vi "wait.vi"(8 "error in (no error)":errorcluster, 10 "wait for":T1, 11 "DL090430TriggeredExperimentController in":refnum<class "ExperimentControllerDL090430DAQmxTriggered.lvclass">) -> (0 "error out":errorcluster, 2 "experiment finished?":bool, 3 "DL090430TriggeredExperimentController out":refnum<class "ExperimentControllerDL090430DAQmxTriggered.lvclass">)   [LabVIEW 2010, in "ExperimentControllerDL090430DAQmxTriggered.lvclass"]
uses:
  ExperimentControllerDL090430DAQmxTriggered.lvclass
  wait_for_enum.ctl
  ExperimentControllerDL090430DAQmxTriggered.lvclass/ExperimentControllerDL090430DAQmxTriggered.ctl
  <vilib>/DAQmx/read.llb/DAQmx Read (Analog DBL 1Chan 1Samp).vi
  <vilib>/DAQmx/configure/trigger.llb/DAQmx Start Trigger (Digital Edge).vi
  <vilib>/daqmx/miscellaneous.llb/DAQmx Fill In Error Info.vi
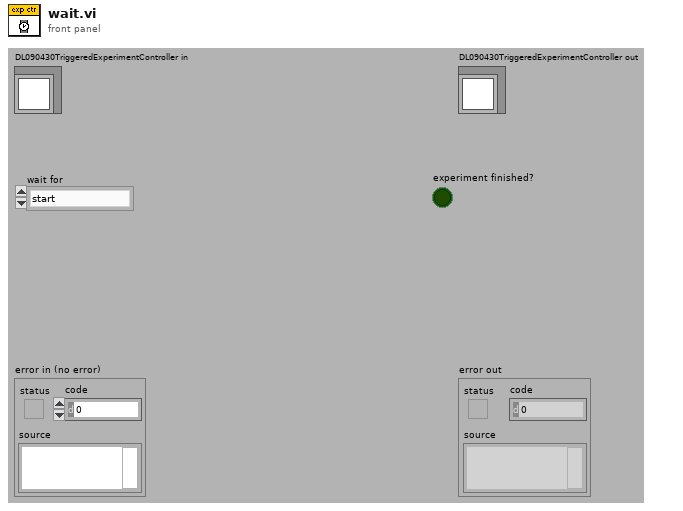
[diagram p1: front panel]
types:
  T1 = typedef "ExperimentControllerDL090430DAQmxTriggered.lvclass/wait_for_enum.ctl" = enum16{"start", "stop"}
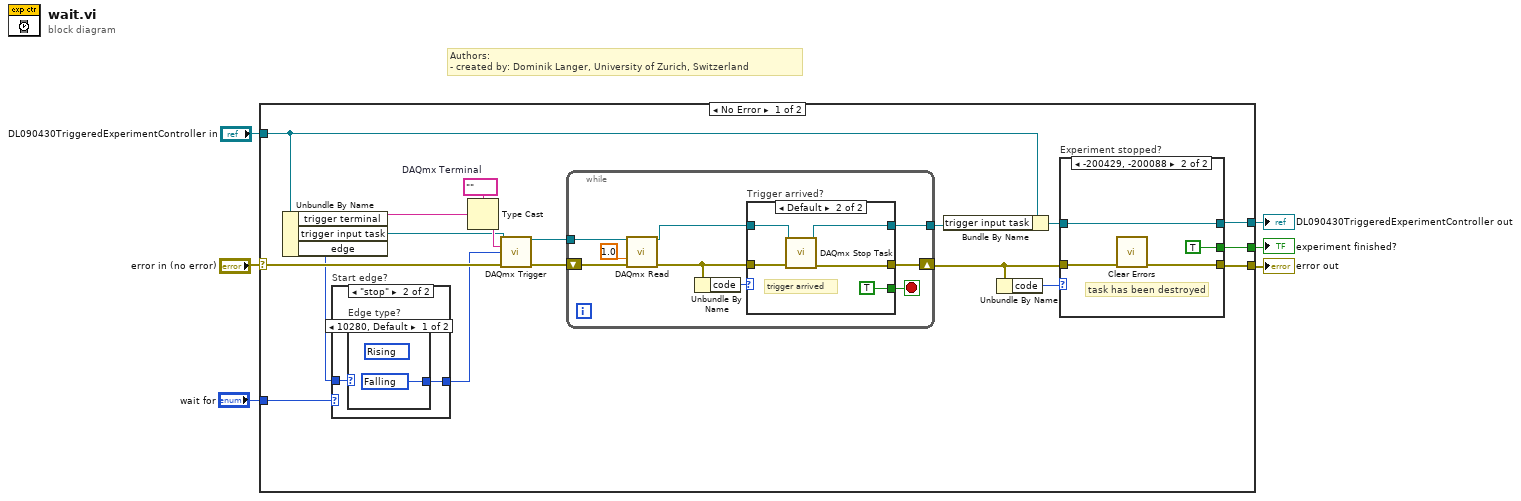
[diagram p0: block diagram]
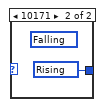
[diagram p3: hidden frame]
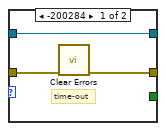
[diagram p5: hidden frame]
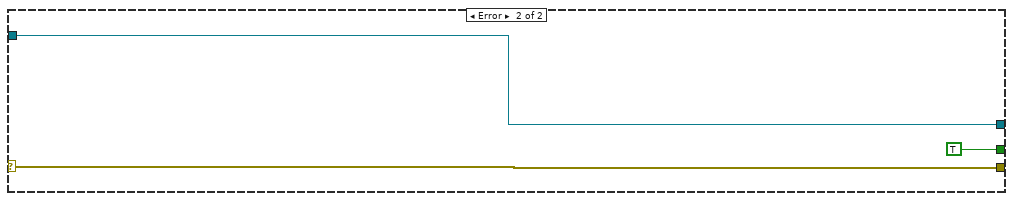
[diagram p6: hidden frame]
diagram:
  # "Authors: \n- created by: Dominik Langer, University of Zurich, Switzerland"
  n1 = case shown="No Error" "error in (no error)" {
    selector: "error in (no error)" -> [w12 w55]
    tunnel: [w21 w55] -> w5
    tunnel: [w19 w54] -> w3
    tunnel: "DL090430TriggeredExperimentController in" -> [w24 w54]
    tunnel: [w17 TRUE] -> w2
    tunnel: "wait for" -> [w9 _]
    frame No Error {
      w16 = tag ""  # DAQmx Terminal
      n2 = Unbundle By Name(w24) -> ("trigger terminal"=w10:string, "trigger input task"=w14:refnum<k21>, "edge"=w8:i32)
      n3 = case "Start edge?" shown="\"stop\"" w9 {
        tunnel: w8 -> [w25 w27]
        tunnel: [w25 w26] -> w7
        frame "start", Default {
        }
        frame "stop" {
          n4 = case "Edge type?" shown="10280, Default" w27 {
            tunnel: [w28 w29] -> w26
            frame 10280, Default {
              w28 = 10171 items=["Rising"=10280, "Falling"=10171] ("edge")
              (unwired) 10280 items=["Rising"=10280, "Falling"=10171] ("edge")
            }
            frame 10171 {
              w29 = 10280 items=["Rising"=10280, "Falling"=10171] ("edge")
              (unwired) 10171 items=["Rising"=10280, "Falling"=10171] ("edge")
            }
          }
        }
      }
      n5 = Type Cast(type=w16, x=w10) -> (*(type *) &x=w15:tag)
      n6 = call-poly <vilib>:"DAQmx Trigger.vi"("task/channels in"=w14, "source"=w15, "edge"=w7, "error in"=w12) -> ("task out"=w13:refnum<k21>, "error out"=w11:errorcluster)  [unwired: 10 out]
      n7 = while {
        tunnel: w13 -> [w43]
        shift-right: [w40] -> w22
        shift-left: w11 -> [w44]
        tunnel: [w38] -> w23
        stop <- w36 stop-if-true
        n8 = call-poly <vilib>:"DAQmx Read.vi"("task/channels in"=w43, "timeout"=1.0, "error in"=w44) -> ("task out"=w39:refnum<k21>, "error out"=w41:errorcluster)  [unwired: 11 out]
        n9 = Unbundle By Name(w41) -> ("code"=w37:i32)
        n10 = case "Trigger arrived?" shown="Default" w37 {
          tunnel: w41 -> [w47 w52]
          tunnel: [w46 w51] -> w40
          tunnel: w39 -> [w45 w50]
          tunnel: [w45 w49] -> w38
          tunnel: [_ TRUE] -> w36
          frame -200284 {
            # "time-out"
            n11 = call <vilib>:"Clear Errors.vi"("error in (no error)"=w47) -> ("error out"=w46:errorcluster)  [unwired: 6 out]
          }
          frame Default {
            # "trigger arrived"
            n12 = call <vilib>:"DAQmx Stop Task.vi"("task/channels in"=w50, "error in"=w52) -> ("task out"=w49:refnum<k21>, "error out"=w51:errorcluster)  [unwired: 12 out]
          }
        }
      }
      n13 = Bundle By Name(cluster=w24, "trigger input task"=w23) -> (w20:refnum<class "ExperimentControllerDL090430DAQmxTriggered.lvclass">)
      n14 = Unbundle By Name(w22) -> ("code"=w18:i32)
      n15 = case "Experiment stopped?" shown="-200429, -200088" w18 {
        tunnel: w22 -> [w31 w35]
        tunnel: [w31 w34] -> w21
        tunnel: w20 -> [w30 w32]
        tunnel: [w30 w32] -> w19
        tunnel: [_ TRUE] -> w17
        frame 0, Default {
        }
        frame -200429, -200088 {
          # "task has been destroyed"
          n16 = call <vilib>:"Clear Errors.vi"("error in (no error)"=w35) -> ("error out"=w34:errorcluster)  [unwired: 6 out]
        }
      }
    }
    frame Error {
    }
  }
  "error out" <- w5
  "DL090430TriggeredExperimentController out" <- w3
  "experiment finished?" <- w2
